vi "9870 Interface DMA (FPGA).vi"() -> ()   [LabVIEW 2012]
uses:
  <vilib>/eio/EIOMethodNode/EIOMethodNode.xnode
  <vilib>/eio/EIOPropertyNode/EIOPropertyNode.xnode
  <vilib>/rvi/DataTransferAndStorage/Container/XNode/niFpgaContainer.xnode
  <vilib>/rvi/interface/RandomDataEmulation/nirviRandomDataFpgaReadWriteTemplate.vi
  <vilib>/rvi/eio/common/nirviEmuTemplatePropertyGet_errors.vi
  <vilib>/rvi/eio/common/nirviEmuTemplatePropertyGet_noerrors.vi
  <vilib>/rvi/eio/common/nirviEmuTemplatePropertySet_errors.vi
  <vilib>/rvi/eio/common/nirviEmuTemplatePropertySet_noerrors.vi
  <vilib>/LabVIEW Targets/FPGA/cRIO/shared/nicrio_ModuleControls/nicrio_cRIO-9871_StopBitsEnum.ctl
  <vilib>/LabVIEW Targets/FPGA/cRIO/shared/nicrio_ModuleControls/nicrio_cRIO-9871_DataBitsEnum.ctl
  <vilib>/LabVIEW Targets/FPGA/cRIO/shared/nicrio_ModuleControls/nicrio_cRIO-9871_FlowControlEnum.ctl
  <vilib>/LabVIEW Targets/FPGA/cRIO/shared/nicrio_ModuleControls/nicrio_cRIO-9871_ParityEnum.ctl
  <vilib>/LabVIEW Targets/FPGA/cRIO/shared/nicrio_ModuleControls/nicrio_cRIO-9871_BaudRateEnum.ctl
  <vilib>/rvi/eio/common/nirviEmuTemplateMethod_errors.vi
panel:
  out "Error Out":errorcluster
  out "error out 4":errorcluster
  out "error out 3":errorcluster
  out "error out 2":errorcluster
  in  "Write Data (FPGA)":bool
  in  "Port To Write (FPGA)":enum8{"0", "1", "2", "3", "4"}(ring)
  in  "Port 1":T6={"Baud Rate"=enum."9600 bps", "Data Bits"=enum."8", "Parity"=enum."None", "Stop Bits"=enum."1", "Flow Control"=enum."None"}
  in  "Port 3":T6={"Baud Rate"=enum."9600 bps", "Data Bits"=enum."8", "Parity"=enum."None", "Stop Bits"=enum."1", "Flow Control"=enum."None"}
  in  "Port 4":T6={"Baud Rate"=enum."9600 bps", "Data Bits"=enum."8", "Parity"=enum."None", "Stop Bits"=enum."1", "Flow Control"=enum."None"}
  in  "Port 2":T6={"Baud Rate"=enum."9600 bps", "Data Bits"=enum."8", "Parity"=enum."None", "Stop Bits"=enum."1", "Flow Control"=enum."None"}
  in  "Bytes to Send":i32
  in  "Timeout (ms)":i32=1
  in  "Update Config":bool
  out "error out 1":errorcluster
  # "Port Read Timeout"
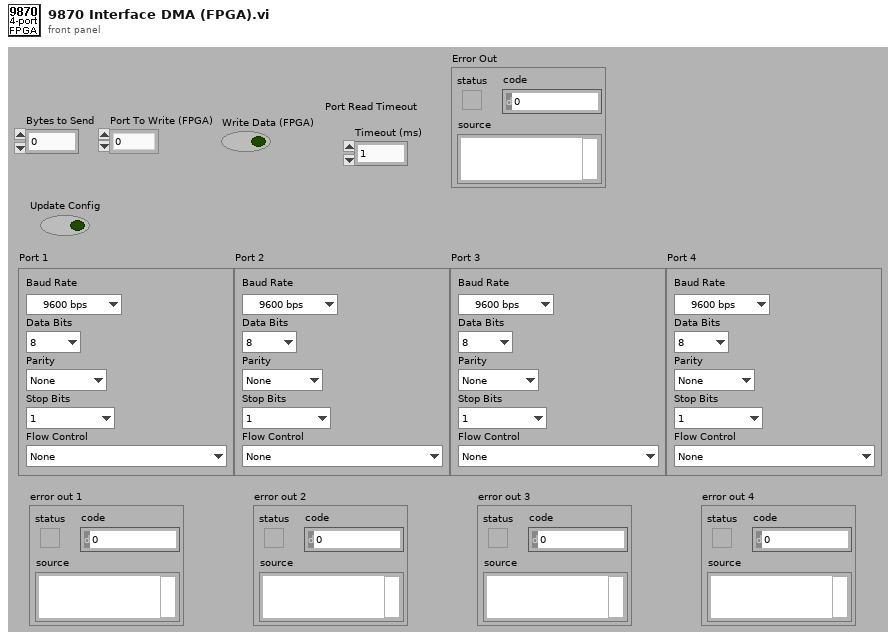
[diagram p1: front panel]
types:
  T1 = typedef "nicrio_cRIO-9871_BaudRateEnum.ctl" = enum16{"75 bps", "110 bps", "134 bps", "150 bps", "300 bps", "600 bps", "1200 bps", "1800 bps", "2400 bps", "4800 bps", "7200 bps", "9600 bps", "14.4 kbps", "19.2 kbps", "28.8 kbps", "38.4 kbps", "57.6 kbps", "115.2 kbps", "230.4 kbps", "460.8 kbps", "921.6 kbps"}
  T2 = typedef "nicrio_cRIO-9871_DataBitsEnum.ctl" = enum8{"5", "6", "7", "8"}
  T3 = typedef "nicrio_cRIO-9871_ParityEnum.ctl" = enum8{"None", "Odd", "Even", "Mark", "Space"}
  T4 = typedef "nicrio_cRIO-9871_StopBitsEnum.ctl" = enum8{"1", "1.5", "2"}
  T5 = typedef "nicrio_cRIO-9871_FlowControlEnum.ctl" = enum8{"None", "Software (XON / XOFF)", "Hardware (RTS / CTS)"}
  T6 = cluster{"Baud Rate":T1, "Data Bits":T2, "Parity":T3, "Stop Bits":T4, "Flow Control":T5}
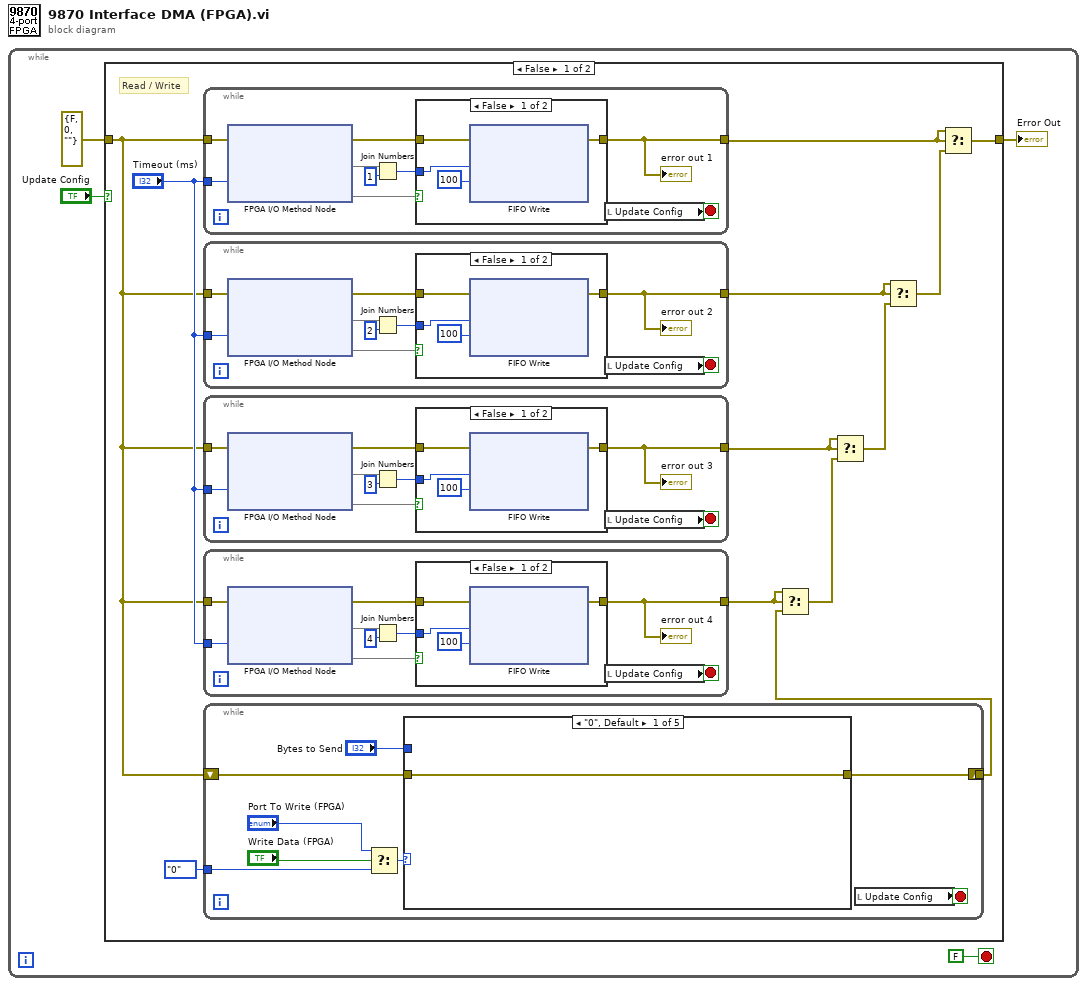
[diagram p0: block diagram]
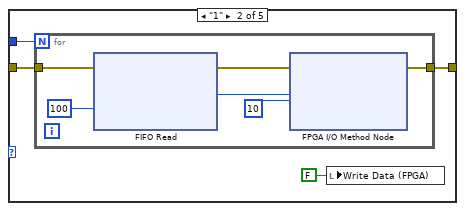
[diagram p5: hidden frame]
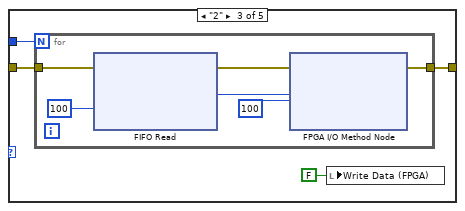
[diagram p6: hidden frame]
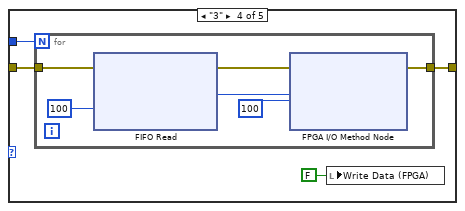
[diagram p7: hidden frame]
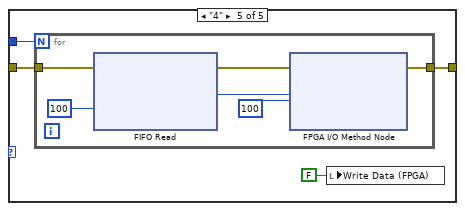
[diagram p8: hidden frame]
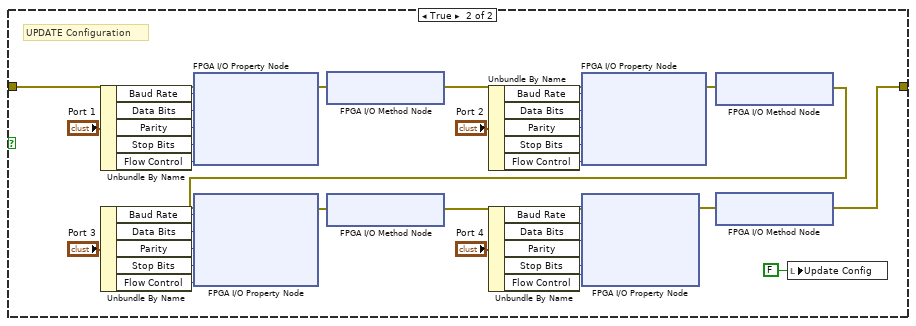
[diagram p10: hidden frame]
diagram:
  n1 = while {
    stop <- FALSE ("Boolean") stop-if-true
    n2 = case shown="False" "Update Config" {
      tunnel: [w8 w122] -> w1
      tunnel: errorcluster {"status"=FALSE, "code"=0, "source"=""} ("error out") -> [w14 w131]
      frame False {
        # "Read / Write"
        n3 = while {
          tunnel: "Timeout (ms)" -> [w111]
          tunnel: w14 -> [w116]
          tunnel: [w108] -> w12
          stop <- w109 stop-if-true
          n4 = xnode "FPGA I/O Method Node"("error in"=w116, "Timeout (ms)"=w111) -> ("error out"=w110:errorcluster, "Data"=w114, "Timed Out"=w115)  [unwired: 1 in, 1 out]
          n5 = Join Numbers(hi=w114, lo=u8 1) -> ((hi.lo)=w112:u16)
          n6 = case shown="False" w115 {
            tunnel: w112 -> [w119 _]
            tunnel: w110 -> [w118 w121]
            tunnel: [w117 w121] -> w108
            frame False {
              n7 = xnode ("FIFO Write")("Element"=w119, "Timeout"=100, "error in (no error)"=w118) -> ("error out"=w117:errorcluster)  [unwired: 1 in, 2 out]
            }
            frame True {
            }
          }
          "error out 1" <- w108
          n8 = local read "Update Config"() -> (w109:bool)
        }
        n9 = while {
          tunnel: "Timeout (ms)" -> [w48]
          tunnel: w14 -> [w53]
          tunnel: [w45] -> w13
          stop <- w46 stop-if-true
          n10 = xnode "FPGA I/O Method Node"("error in"=w53, "Timeout (ms)"=w48) -> ("error out"=w47:errorcluster, "Data"=w51, "Timed Out"=w52)  [unwired: 1 in, 1 out]
          n11 = Join Numbers(hi=w51, lo=u8 2) -> ((hi.lo)=w49:u16)
          n12 = case shown="False" w52 {
            tunnel: w49 -> [w56 _]
            tunnel: w47 -> [w55 w58]
            tunnel: [w54 w58] -> w45
            frame False {
              n13 = xnode ("FIFO Write")("Element"=w56, "Timeout"=100, "error in (no error)"=w55) -> ("error out"=w54:errorcluster)  [unwired: 1 in, 2 out]
            }
            frame True {
            }
          }
          "error out 2" <- w45
          n14 = local read "Update Config"() -> (w46:bool)
        }
        n15 = while {
          tunnel: "Timeout (ms)" -> [w34]
          tunnel: w14 -> [w39]
          tunnel: [w31] -> w11
          stop <- w32 stop-if-true
          n16 = xnode "FPGA I/O Method Node"("error in"=w39, "Timeout (ms)"=w34) -> ("error out"=w33:errorcluster, "Data"=w37, "Timed Out"=w38)  [unwired: 1 in, 1 out]
          n17 = Join Numbers(hi=w37, lo=u8 3) -> ((hi.lo)=w35:u16)
          n18 = case shown="False" w38 {
            tunnel: w35 -> [w42 _]
            tunnel: w33 -> [w41 w44]
            tunnel: [w40 w44] -> w31
            frame False {
              n19 = xnode ("FIFO Write")("Element"=w42, "Timeout"=100, "error in (no error)"=w41) -> ("error out"=w40:errorcluster)  [unwired: 1 in, 2 out]
            }
            frame True {
            }
          }
          "error out 3" <- w31
          n20 = local read "Update Config"() -> (w32:bool)
        }
        n21 = while {
          tunnel: "Timeout (ms)" -> [w20]
          tunnel: w14 -> [w25]
          tunnel: [w17] -> w7
          stop <- w18 stop-if-true
          n22 = xnode "FPGA I/O Method Node"("error in"=w25, "Timeout (ms)"=w20) -> ("error out"=w19:errorcluster, "Data"=w23, "Timed Out"=w24)  [unwired: 1 in, 1 out]
          n23 = Join Numbers(hi=w23, lo=u8 4) -> ((hi.lo)=w21:u16)
          n24 = case shown="False" w24 {
            tunnel: w21 -> [w28 _]
            tunnel: w19 -> [w27 w30]
            tunnel: [w26 w30] -> w17
            frame False {
              n25 = xnode ("FIFO Write")("Element"=w28, "Timeout"=100, "error in (no error)"=w27) -> ("error out"=w26:errorcluster)  [unwired: 1 in, 2 out]
            }
            frame True {
            }
          }
          "error out 4" <- w17
          n26 = local read "Update Config"() -> (w18:bool)
        }
        n27 = while {
          shift-right: [w63] -> w5
          shift-left: w14 -> [w66]
          tunnel: enum8{"0", "1", "2", "3", "4"}."0" ("Port To Write (FPGA) 2") -> [w61]
          tunnel: [w63] -> _
          stop <- w65 stop-if-true
          n28 = Select(t="Port To Write (FPGA)", s="Write Data (FPGA)", f=w61) -> (s? t:f=w60:enum8{"0", "1", "2", "3", "4"})
          n29 = case shown="\"0\", Default" w60 {
            tunnel: w66 -> [w67 w71 w81 w91 w101]
            tunnel: "Bytes to Send" -> [_ w70 w80 w90 w100]
            tunnel: [w67 w69 w79 w89 w99] -> w63
            frame "0", Default {
            }
            frame "1" {
              n30 = for {
                N: w70 -> [_]
                tunnel: w71 -> [w76]
                tunnel: [w72] -> w69
                n31 = xnode ("FIFO Read")("Timeout"=100 ("Timeout (ms)"), "error in (no error)"=w76) -> ("Element"=w77:u8, "error out"=w75:errorcluster)  [unwired: 1 in, 2 out]
                n32 = xnode "FPGA I/O Method Node"("error in"=w75, "Data"=w77, "Timeout (ms)"=10) -> ("error out"=w72:errorcluster)  [unwired: 1 in, 2 out]
              }
              n33 = local write "Write Data (FPGA)"(FALSE ("Write Data (FPGA)")) -> ()
            }
            frame "2" {
              n34 = for {
                N: w80 -> [_]
                tunnel: w81 -> [w86]
                tunnel: [w82] -> w79
                n35 = xnode ("FIFO Read")("Timeout"=100 ("Timeout (ms)"), "error in (no error)"=w86) -> ("Element"=w87:u8, "error out"=w85:errorcluster)  [unwired: 1 in, 2 out]
                n36 = xnode "FPGA I/O Method Node"("error in"=w85, "Data"=w87, "Timeout (ms)"=100) -> ("error out"=w82:errorcluster)  [unwired: 1 in, 2 out]
              }
              n37 = local write "Write Data (FPGA)"(FALSE ("Write Data (FPGA)")) -> ()
            }
            frame "3" {
              n38 = for {
                N: w90 -> [_]
                tunnel: w91 -> [w96]
                tunnel: [w92] -> w89
                n39 = xnode ("FIFO Read")("Timeout"=100 ("Timeout (ms)"), "error in (no error)"=w96) -> ("Element"=w97:u8, "error out"=w95:errorcluster)  [unwired: 1 in, 2 out]
                n40 = xnode "FPGA I/O Method Node"("error in"=w95, "Data"=w97, "Timeout (ms)"=100) -> ("error out"=w92:errorcluster)  [unwired: 1 in, 2 out]
              }
              n41 = local write "Write Data (FPGA)"(FALSE ("Write Data (FPGA)")) -> ()
            }
            frame "4" {
              n42 = for {
                N: w100 -> [_]
                tunnel: w101 -> [w106]
                tunnel: [w102] -> w99
                n43 = xnode ("FIFO Read")("Timeout"=100 ("Timeout (ms)"), "error in (no error)"=w106) -> ("Element"=w107:u8, "error out"=w105:errorcluster)  [unwired: 1 in, 2 out]
                n44 = xnode "FPGA I/O Method Node"("error in"=w105, "Data"=w107, "Timeout (ms)"=100) -> ("error out"=w102:errorcluster)  [unwired: 1 in, 2 out]
              }
              n45 = local write "Write Data (FPGA)"(FALSE ("Write Data (FPGA)")) -> ()
            }
          }
          n46 = local read "Update Config"() -> (w65:bool)
        }
        n47 = Select(t=w7, s=w7, f=w5) -> (s? t:f=w6:errorcluster)
        n48 = Select(t=w11, s=w11, f=w6) -> (s? t:f=w9:errorcluster)
        n49 = Select(t=w13, s=w13, f=w9) -> (s? t:f=w10:errorcluster)
        n50 = Select(t=w12, s=w12, f=w10) -> (s? t:f=w8:errorcluster)
      }
      frame True {
        # "UPDATE Configuration"
        n51 = Unbundle By Name("Port 1") -> ("Baud Rate"=w154:T1, "Data Bits"=w153:T2, "Parity"=w152:T3, "Stop Bits"=w151:T4, "Flow Control"=w150:T5)
        n52 = Unbundle By Name("Port 3") -> ("Baud Rate"=w138:T1, "Data Bits"=w139:T2, "Parity"=w140:T3, "Stop Bits"=w141:T4, "Flow Control"=w142:T5)
        n53 = xnode "FPGA I/O Property Node"("error in"=w131, "Baud Rate"=w154, "Data Bits"=w153, "Parity"=w152, "Stop Bits"=w151, "Flow Control"=w150) -> ("error out"=w129:errorcluster)  [unwired: 1 in, 1 out]
        n54 = xnode "FPGA I/O Method Node"("error in"=w129) -> ("error out"=w128:errorcluster)  [unwired: 1 in, 1 out]
        n55 = Unbundle By Name("Port 2") -> ("Baud Rate"=w148:T1, "Data Bits"=w147:T2, "Parity"=w146:T3, "Stop Bits"=w145:T4, "Flow Control"=w144:T5)
        n56 = Unbundle By Name("Port 4") -> ("Baud Rate"=w132:T1, "Data Bits"=w133:T2, "Parity"=w134:T3, "Stop Bits"=w135:T4, "Flow Control"=w136:T5)
        n57 = xnode "FPGA I/O Property Node"("error in"=w128, "Baud Rate"=w148, "Data Bits"=w147, "Parity"=w146, "Stop Bits"=w145, "Flow Control"=w144) -> ("error out"=w127:errorcluster)  [unwired: 1 in, 1 out]
        n58 = xnode "FPGA I/O Method Node"("error in"=w127) -> ("error out"=w126:errorcluster)  [unwired: 1 in, 1 out]
        n59 = xnode "FPGA I/O Property Node"("error in"=w126, "Baud Rate"=w138, "Data Bits"=w139, "Parity"=w140, "Stop Bits"=w141, "Flow Control"=w142) -> ("error out"=w125:errorcluster)  [unwired: 1 in, 1 out]
        n60 = xnode "FPGA I/O Method Node"("error in"=w125) -> ("error out"=w124:errorcluster)  [unwired: 1 in, 1 out]
        n61 = xnode "FPGA I/O Property Node"("error in"=w124, "Baud Rate"=w132, "Data Bits"=w133, "Parity"=w134, "Stop Bits"=w135, "Flow Control"=w136) -> ("error out"=w123:errorcluster)  [unwired: 1 in, 1 out]
        n62 = xnode "FPGA I/O Method Node"("error in"=w123) -> ("error out"=w122:errorcluster)  [unwired: 1 in, 1 out]
        n63 = local write "Update Config"(FALSE ("Update Config")) -> ()
      }
    }
    "Error Out" <- w1
  }
